vi "anda_dist.vi"() -> ()   [LabVIEW 2016]
uses:
  <vilib>/NXT/Subs/LVHSConnector.ctl
  <vilib>/NXT/LegoClasses/BrickReference/BrickReference.lvclass
  <vilib>/NXT/Block Support/NXT_OutputPort.ctl
  <vilib>/NXT/Dual Mode Library/Motors/ResetMotor.vi
  <vilib>/NXT/Dual Mode Library/Motors/Rotation.vi
  <vilib>/NXT/Dual Mode Library/Display/drawNumber.vi
  <vilib>/NXT/NXTIO Xnodes/AddressXNode/NXTIOAddress.xnode
panel:
  in  "dist (rad)":i32
  out "Angle of Rotation":i32
  in  "NXT/EV3":T1
  out "NXT/EV3 2":T1
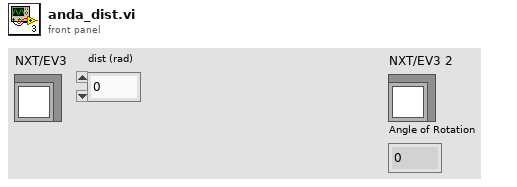
[diagram p1: front panel]
types:
  T1 = typedef "LVHSConnector.ctl" = refnum<class "BrickReference.lvclass">
  T2 = typedef "NXT_OutputPort.ctl" = u8
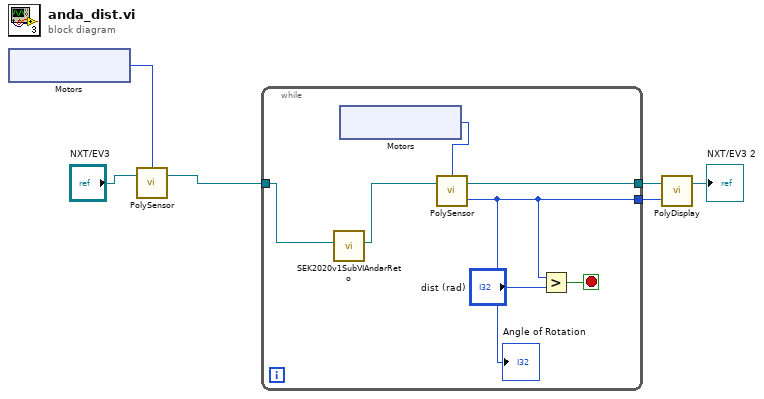
[diagram p0: block diagram]
diagram:
  n1 = xnode "Motors"() -> ("Motor"=w2:T2)
  n2 = call-poly <vilib>:"PolySensor.vi"("NXT/EV3"="NXT/EV3", "Port (All Ports)"=w2) -> ("NXT/EV3"=w1:T1)  [unwired: 2 out]
  n3 = while {
    tunnel: w1 -> [w9]
    tunnel: [w13] -> w4
    tunnel: [w12] -> w5
    stop <- w10 stop-if-true
    n4 = call "SEK2020v1SubVIAndarReto.vi"("NXT/EV3"=w9) -> ("NXT/EV3 2"=w8:T1)  [unwired: 9 in]
    n5 = xnode "Motors"() -> ("Motor"=w7:T2)
    n6 = call-poly <vilib>:"PolySensor.vi"("NXT/EV3"=w8, "Port (Port A)"=w7) -> ("Angle of Rotation"=w12:i32, "NXT/EV3"=w13:T1)  [unwired: 1 out]
    "Angle of Rotation" <- w12
    n7 = Greater?(x=w12, y="dist (rad)") -> (0:w10:bool)
  }
  n8 = call-poly <vilib>:"PolyDisplay.vi"("number"=w5, "NXT/EV3"=w4) -> ("NXT/EV3"=→"NXT/EV3 2":T1)  [unwired: 2 in]
